vi "test send cmd.vi"() -> ()   [LabVIEW 2016]
panel:
  out "Response":string
  out "switch info":string
  out "error code":string
  out "result":string
  out "serial number":string
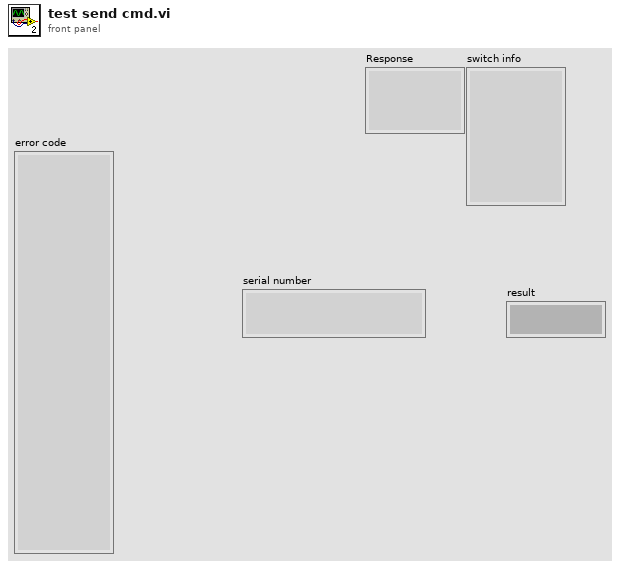
[diagram p1: front panel]
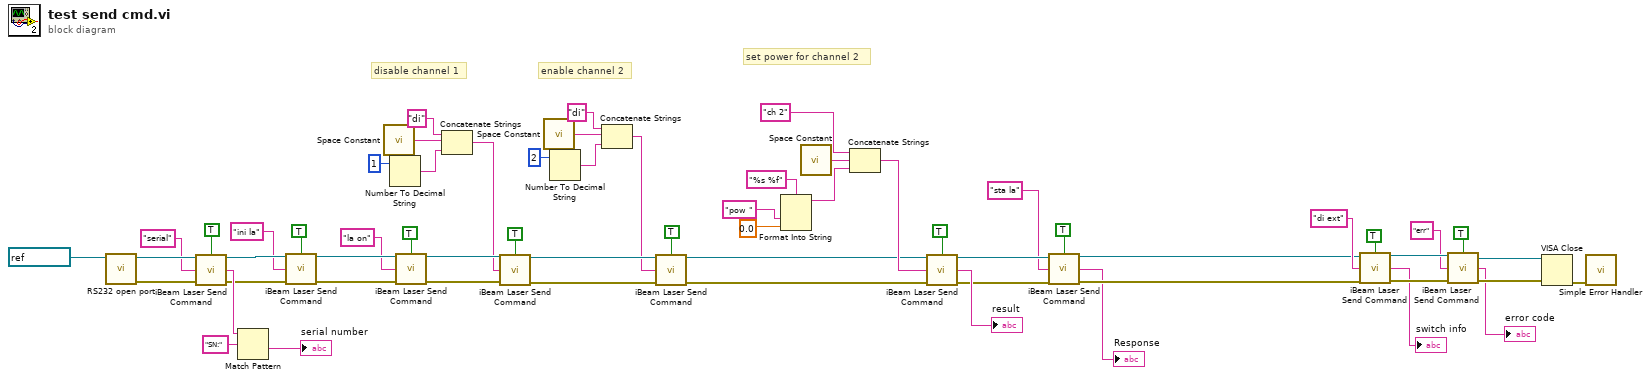
[diagram p0: block diagram]
diagram:
  # "set power for channel 2"
  # "enable channel 2"
  # "disable channel 1"
  n1 = call "RS232 open port.vi"("VISA resource name"=refnum<visa-resource-name> "COM4") -> ("error out"=w27:errorcluster, "dup VISA resource name"=w61:refnum<visa-resource-name>)  [unwired: 5 in]
  n2 = call "iBeam Laser Send Command.vi"("VISA Ref"=w61, "Wait for Reply?"=TRUE, "Command"="serial" ("command"), "Error In"=w27) -> ("VISA Ref Out"=w56:refnum<visa-resource-name>, "Response"=w26:string, "Error Out"=w25:errorcluster)  [unwired: 9 in]
  n3 = Match Pattern(string=w26, regular expression="SN:") -> (after substring=→"serial number":string)  [unwired: 1 in, 3 out]
  n4 = call "iBeam Laser Send Command.vi"("VISA Ref"=w56, "Wait for Reply?"=TRUE, "Command"="ini la" ("command"), "Error In"=w25) -> ("VISA Ref Out"=w54:refnum<visa-resource-name>, "Error Out"=w53:errorcluster)  [unwired: 9 in, 1 out]
  n5 = call <vilib>:"Space Constant.vi"() -> ("String"=w47:string)
  n6 = Number To Decimal String(number=1) -> (decimal integer string=w46:string)  [unwired: 1 in]
  n7 = call "iBeam Laser Send Command.vi"("VISA Ref"=w54, "Wait for Reply?"=TRUE, "Command"="la on" ("command"), "Error In"=w53) -> ("VISA Ref Out"=w51:refnum<visa-resource-name>, "Error Out"=w50:errorcluster)  [unwired: 9 in, 1 out]
  n8 = Concatenate Strings("di" ("string"), w47, w46) -> (w45:string)
  n9 = call "iBeam Laser Send Command.vi"("VISA Ref"=w51, "Wait for Reply?"=TRUE, "Command"=w45, "Error In"=w50) -> ("VISA Ref Out"=w44:refnum<visa-resource-name>, "Error Out"=w43:errorcluster)  [unwired: 9 in, 1 out]
  n10 = call <vilib>:"Space Constant.vi"() -> ("String"=w40:string)
  n11 = Number To Decimal String(number=2) -> (decimal integer string=w39:string)  [unwired: 1 in]
  n12 = Concatenate Strings("di" ("string"), w40, w39) -> (w38:string)
  n13 = call "iBeam Laser Send Command.vi"("VISA Ref"=w44, "Wait for Reply?"=TRUE, "Command"=w38, "Error In"=w43) -> ("VISA Ref Out"=w31:refnum<visa-resource-name>, "Error Out"=w30:errorcluster)  [unwired: 9 in, 1 out]
  n14 = Format Into String(format string="%s %f", "pow " ("string"), sgl 0.0) -> (resulting string=w33:string)  [unwired: 2 in, 1 out]
  n15 = call <vilib>:"Space Constant.vi"() -> ("String"=w34:string)
  n16 = Concatenate Strings("ch 2" ("string"), w34, w33) -> (w32:string)
  n17 = call "iBeam Laser Send Command.vi"("VISA Ref"=w31, "Wait for Reply?"=TRUE, "Command"=w32, "Error In"=w30) -> ("VISA Ref Out"=w18:refnum<visa-resource-name>, "Response"=→"result":string, "Error Out"=w17:errorcluster)  [unwired: 9 in]
  n18 = call "iBeam Laser Send Command.vi"("VISA Ref"=w18, "Wait for Reply?"=TRUE, "Command"="sta la", "Error In"=w17) -> ("VISA Ref Out"=w4:refnum<visa-resource-name>, "Response"=→"Response":string, "Error Out"=w3:errorcluster)  [unwired: 9 in]
  n19 = call "iBeam Laser Send Command.vi"("VISA Ref"=w4, "Wait for Reply?"=TRUE, "Command"="di ext", "Error In"=w3) -> ("VISA Ref Out"=w13:refnum<visa-resource-name>, "Response"=→"switch info":string, "Error Out"=w12:errorcluster)  [unwired: 9 in]
  n20 = call "iBeam Laser Send Command.vi"("VISA Ref"=w13, "Wait for Reply?"=TRUE, "Command"="err", "Error In"=w12) -> ("VISA Ref Out"=w10:refnum<visa-resource-name>, "Response"=→"error code":string, "Error Out"=w11:errorcluster)  [unwired: 9 in]
  n21 = VISA Close(VISA resource name=w10, error in (no error)=w11) -> (error out=w57:errorcluster)
  n22 = call <vilib>:"Simple Error Handler.vi"("error in (no error)"=w57) -> ()  [unwired: 4 in, 5 out]
